vi "LVClass_WavefrontCorrector Get Current Preferences.vi"(0 "WavefrontCorrector in":refnum<class "WavefrontCorrector.lvclass">, 11 "error in (no error)":errorcluster) -> (4 "WavefrontCorrector out":refnum<class "WavefrontCorrector.lvclass">, 6 "sleep_after_movement":i32, 8 "Mirror preferences.Wavefront Corrector State":T1[](array[typedef]), 15 "error out":errorcluster)   [LabVIEW 2020, in "WavefrontCorrector.lvclass"]
doc: "Get current preferences.\n\n--------------------------------------------------------------------------------\n\n<B>correctorIn </B> : WavefrontCorrector object.\n<B>correctorOut </B> : WavefrontCorrector object.\n<B>sleep_after_movement </B> : WavefrontCorrector preferences : Time to stabilization (ms).\n<B>min </B> : WavefrontCorrector preferences : lowest command value.\n<B>max </B> : WavefrontCorrector preferences : highest command value.\n<B>validity </B> : WavefrontCorrector preferences : status.\n<B>fixed_values </B> : WavefrontCorrector preferences : fixed positions.\n<B>ErrorIn </B> : Error\n<B>ErrorOut </B> : Error\n\n--------------------------------------------------------------------------------"
uses:
  WavefrontCorrector.lvclass
  Wavefront Corrector states - ONE.ctl
  WavefrontCorrector.lvclass/WavefrontCorrector.ctl
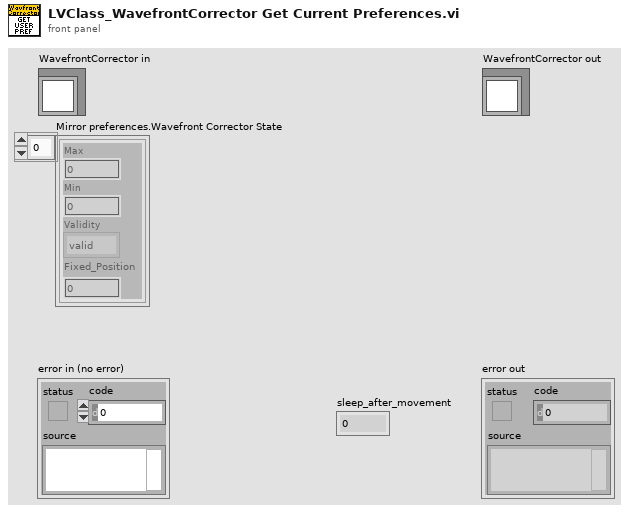
[diagram p1: front panel]
types:
  T1 = typedef "Wavefront Corrector states - ONE.ctl" = cluster{"Max":sgl, "Min":sgl, "Validity":enum16{"valid", "fixed", "invalid"}, "Fixed_Position":sgl}
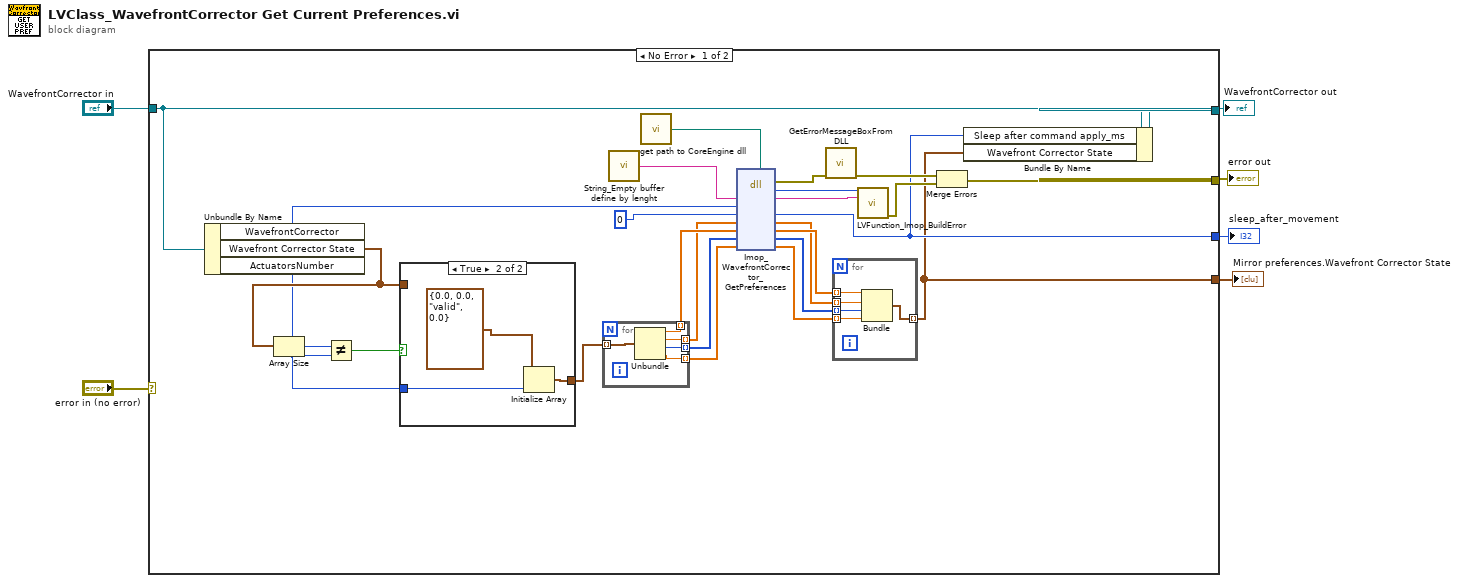
[diagram p0: block diagram]
diagram:
  n1 = case shown="No Error" "error in (no error)" {
    selector: "error in (no error)" -> [_ w49]
    tunnel: [w26 w49] -> w3
    tunnel: [w11 w48] -> w4
    tunnel: "WavefrontCorrector in" -> [w12 w48]
    tunnel: [w8 _] -> w2
    tunnel: [w7 _] -> w1
    frame No Error {
      n2 = Unbundle By Name(w12) -> ("WavefrontCorrector"=w20:i32, "Wavefront Corrector State"=w16:T1[], "ActuatorsNumber"=w10:i32)
      n3 = Array Size(array=w16) -> (size(s)=w18:i32)
      n4 = Not Equal?(x=w18, y=w10) -> (x != y?=w19:bool)
      n5 = case shown="True" w19 {
        tunnel: [w39 w42] -> w9
        tunnel: w10 -> [_ w41]
        tunnel: w16 -> [w39 _]
        frame False {
        }
        frame True {
          n6 = Initialize Array(T1 {"Max"=0.0, "Min"=0.0, "Validity"=enum."valid", "Fixed_Position"=0.0} ("Actuator state"), w41) -> (w42:T1[])
        }
      }
      n7 = for {
        tunnel: [w38] -> w17 mode=indexing
        tunnel: [w37] -> w15 mode=indexing
        tunnel: [w36] -> w14 mode=indexing
        tunnel: [w35] -> w13 mode=indexing
        tunnel: w9 -> [w34] mode=indexing
        n8 = Unbundle(w34) -> ("Max"=w38:sgl, "Min"=w37:sgl, "Validity"=w36:enum16{"valid", "fixed", "invalid"}, "Fixed_Position"=w35:sgl)
      }
      n9 = call "String_Empty buffer define by lenght.vi"() -> ("Empty buffer"=w31:string)  [unwired: 1 in]
      n10 = call "get path to CoreEngine dll.vi"() -> ("path to c_interface_vc100.dll"=w30:path)  [unwired: 12 in, 3 out]
      n11 = dll-call lib="D:/soft/HASO_v3/SVN_trunk/ImOpCoreEngine4_LV2011/DLLs/c_interface_vc100.dll" fn="Imop_WavefrontCorrector_GetPreferences"(path in=w30, "message"=w31, "WavefrontCorrection"=w20, "sleep_after_movement"=0, "min"=w15, "max"=w17, "validity"=w14, "fixed_value"=w13) -> (error out=w29:errorcluster, "return type"=w33:i32, "message"=w32:string, "sleep_after_movement"=w8:i32, "min"=w24:sgl[], "max"=w25:sgl[], "validity"=w23:i32[], "fixed_value"=w22:sgl[])  [unwired: 3 in, 1 out]
      n12 = call "GetErrorMessageBoxFromDLL.vi"("error IN"=w29) -> ("error OUT"=w28:errorcluster)  [unwired: 10 in]
      n13 = for {
        tunnel: w25 -> [w47] mode=indexing
        tunnel: w24 -> [w46] mode=indexing
        tunnel: w23 -> [w45] mode=indexing
        tunnel: w22 -> [w44] mode=indexing
        tunnel: [w43] -> w7 mode=indexing
        n14 = Bundle(w47, w46, w45, w44) -> (w43:cluster{sgl, sgl, i32, sgl})  [unwired: 1 in]
      }
      n15 = call "LVFunction_Imop_BuildError.vi"("code"=w33, "String to Prepend to source (\"\")"=w32) -> ("error out"=w27:errorcluster)  [unwired: 13 in]
      n16 = Merge Errors(w28, w27) -> (w26:errorcluster)
      n17 = Bundle By Name(cluster=w12, "Sleep after command apply_ms"=w8, "Wavefront Corrector State"=w7) -> (w11:refnum<class "WavefrontCorrector.lvclass">)
    }
    frame Error {
    }
  }
  "error out" <- w3
  "WavefrontCorrector out" <- w4
  "sleep_after_movement" <- w2
  "Mirror preferences.Wavefront Corrector State" <- w1
